vi "stopFGV.vi"(10 "stop?":bool, 11 "Enum":T1) -> (2 "stop?":bool)   [LabVIEW 2017]
uses:
  TypeDefs/basicFGVControl.ctl
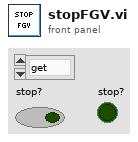
[diagram p1: front panel]
types:
  T1 = typedef "basicFGVControl.ctl" = enum16{"get", "set"}
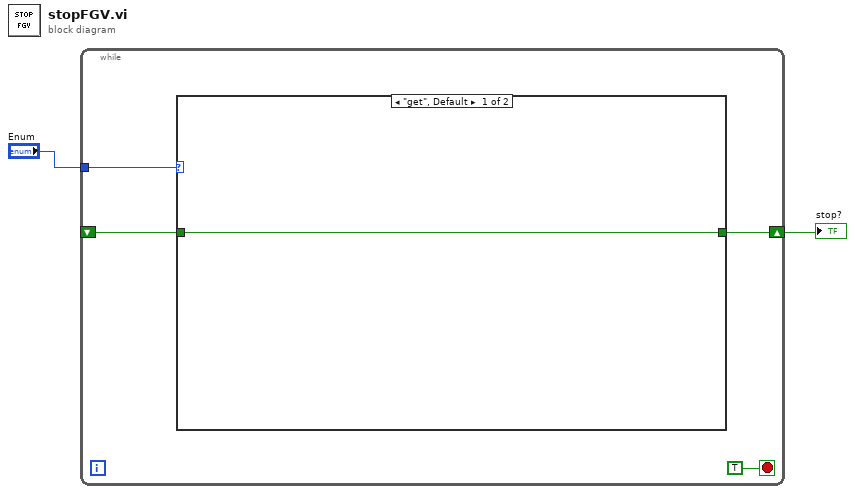
[diagram p0: block diagram]
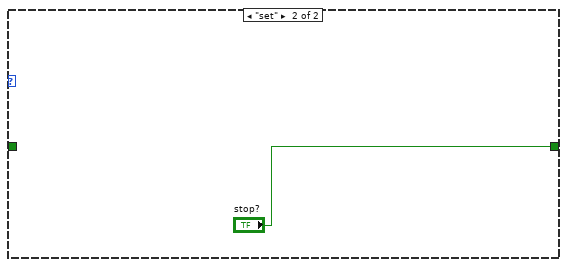
[diagram p2: hidden frame]
diagram:
  n1 = while {
    tunnel: "Enum" -> [w5]
    shift-right: [w4] -> w1
    shift-left: _ -> [w3]
    stop <- TRUE stop-if-true
    n2 = case shown="\"get\", Default" w5 {
      tunnel: [w7 "stop?"] -> w4
      tunnel: w3 -> [w7 _]
      frame "get", Default {
      }
      frame "set" {
      }
    }
  }
  "stop?" <- w1
